vi "Configure.vi"(8 "error in (no error)":errorcluster, 10 "Config":T1[](array[typedef]), 11 "Device in":refnum<class "Device.lvclass">) -> (0 "error out":errorcluster, 3 "Device out":refnum<class "Device.lvclass">)   [LabVIEW 2020, in "HAL.lvlib" / "Device.lvclass"]
uses:
  Device.lvclass
  Config Item.ctl
  Device State.ctl
  Device.lvclass/Device.ctl
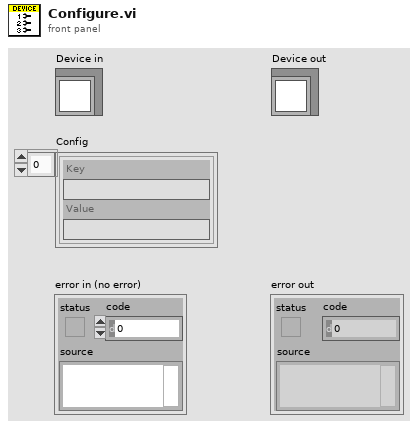
[diagram p1: front panel]
types:
  T1 = typedef "HAL.lvlib/Device.lvclass/Config Item.ctl" = cluster{"Key":string, "Value":string}
  T2 = typedef "HAL.lvlib/Device.lvclass/Device State.ctl" = enum16{"Uninitialized", "Initialized", "Ready", "Running", "Error"}
  T3 = typedef "HAL.lvlib/Device.lvclass/Ref Data.ctl" = cluster{"Config Keys":string[], "Config Values":string[], "Cal Expires":timestamp, "Name":string, "Comment":string, "State":T2, "Error":errorcluster}
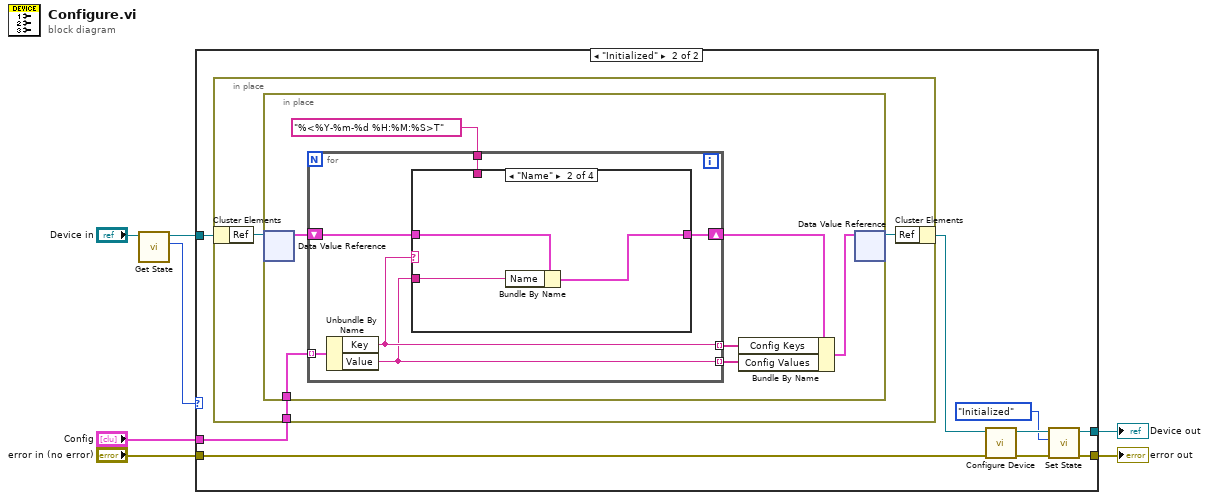
[diagram p0: block diagram]
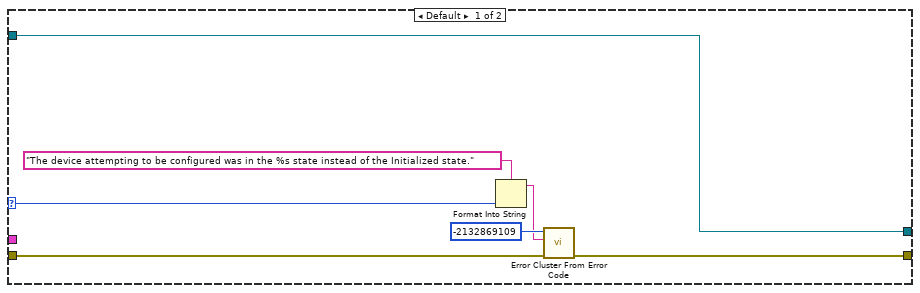
[diagram p2: hidden frame]
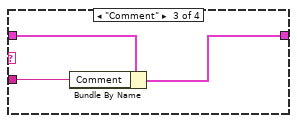
[diagram p4: hidden frame]
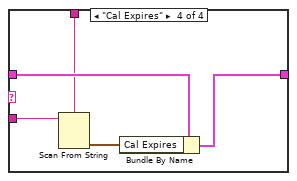
[diagram p5: hidden frame]
diagram:
  n1 = call "Get State.vi"("Device in"="Device in") -> ("Device State"=w2:T2, "Device out"=w1:refnum<class "Device.lvclass">)  [unwired: 8 in, 1 out]
  n2 = case shown="\"Initialized\"" w2 {
    selector: w2 -> [w11 _]
    tunnel: "error in (no error)" -> [w14 w23]
    tunnel: "Config" -> [_ w22]
    tunnel: [w8 w18] -> w5
    tunnel: [w9 w17] -> w4
    tunnel: w1 -> [w8 w15]
    frame Default {
      n3 = Format Into String(format string="The device attempting to be configured was in the %s state instead of the Initialized state." ("error message (\"\")"), w11) -> (resulting string=w10:string)  [unwired: 2 in, 1 out]
      n4 = call <vilib>:"Error Cluster From Error Code.vi"("error in (no error)"=w14, "error message (\"\")"=w10, "error code (0)"=-2132869109) -> ("error out"=w9:errorcluster)  [unwired: 6 in]
    }
    frame "Initialized" {
      n5 = in-place {
        in-place-border: w22 -> [w26]
        n6 = in-place-cluster #1(w15) -> ("Ref"=w25:refnum<data-value>)
        n7 = in-place {
          in-place-border: w26 -> [w33]
          n8 = in-place-dvr #2(w25) -> (w27:T3)  [unwired: 1 out]
          n9 = for {
            shift-right: [w35] -> w32
            shift-left: w27 -> [w36]
            tunnel: w33 -> [w39] mode=indexing
            tunnel: [w37] -> w30 mode=indexing
            tunnel: [w38] -> w31 mode=indexing
            tunnel: "%<%Y-%m-%d %H:%M:%S>T" ("format string") -> [w34]
            n10 = Unbundle By Name(w39) -> ("Key"=w38:string, "Value"=w37:string)
            n11 = case shown="\"Name\"" w38 {
              tunnel: w37 -> [_ w42 w45 w49]
              tunnel: w36 -> [w40 w43 w46 w51]
              tunnel: [w40 w41 w44 w50] -> w35
              tunnel: w34 -> [_ _ _ w48]
              frame Default {
              }
              frame "Name" {
                n12 = Bundle By Name(cluster=w43, "Name"=w42) -> (w41:T3)
              }
              frame "Comment" {
                n13 = Bundle By Name(cluster=w46, "Comment"=w45) -> (w44:T3)
              }
              frame "Cal Expires" {
                n14 = Scan From String(format string=w48, input string=w49) -> (output 1=w47:timestamp)  [unwired: 3 in, 3 out]
                n15 = Bundle By Name(cluster=w51, "Cal Expires"=w47) -> (w50:T3)
              }
            }
          }
          n16 = Bundle By Name(cluster=w32, "Config Keys"=w31, "Config Values"=w30) -> (w28:T3)
          n17 = in-place-dvr #2(w28) -> (w24:refnum<data-value>)  [unwired: 1 out]
        }
        n18 = in-place-cluster #1("Ref"=w24) -> (w16:refnum<class "Device.lvclass">)
      }
      n19 = call-dynamic "Configure Device.vi"("error in (no error)"=w23, "Device in"=w16) -> ("error out"=w20:errorcluster, "Device out"=w21:refnum<class "Device.lvclass">)  [unwired: 8 in]
      n20 = call "Set State.vi"("error in (no error)"=w20, "Device State"=Device_State."Initialized", "Device in"=w21) -> ("error out"=w17:errorcluster, "Device out"=w18:refnum<class "Device.lvclass">)  [unwired: 7 in]
    }
  }
  "error out" <- w4
  "Device out" <- w5
